vi "Filter for Classes.vi"(11 "rename data":T2) -> (1 "found classes?":bool, 3 "renamed classes":T1[](array[typedef]))   [LabVIEW 2021, in "MeasurementService Editor.lvlib"]
uses:
  MeasurementService Editor.lvlib
  Rename Refactor Data.ctl
  Rename Refactor Mapping Info.ctl
  Rename String Mapping.ctl
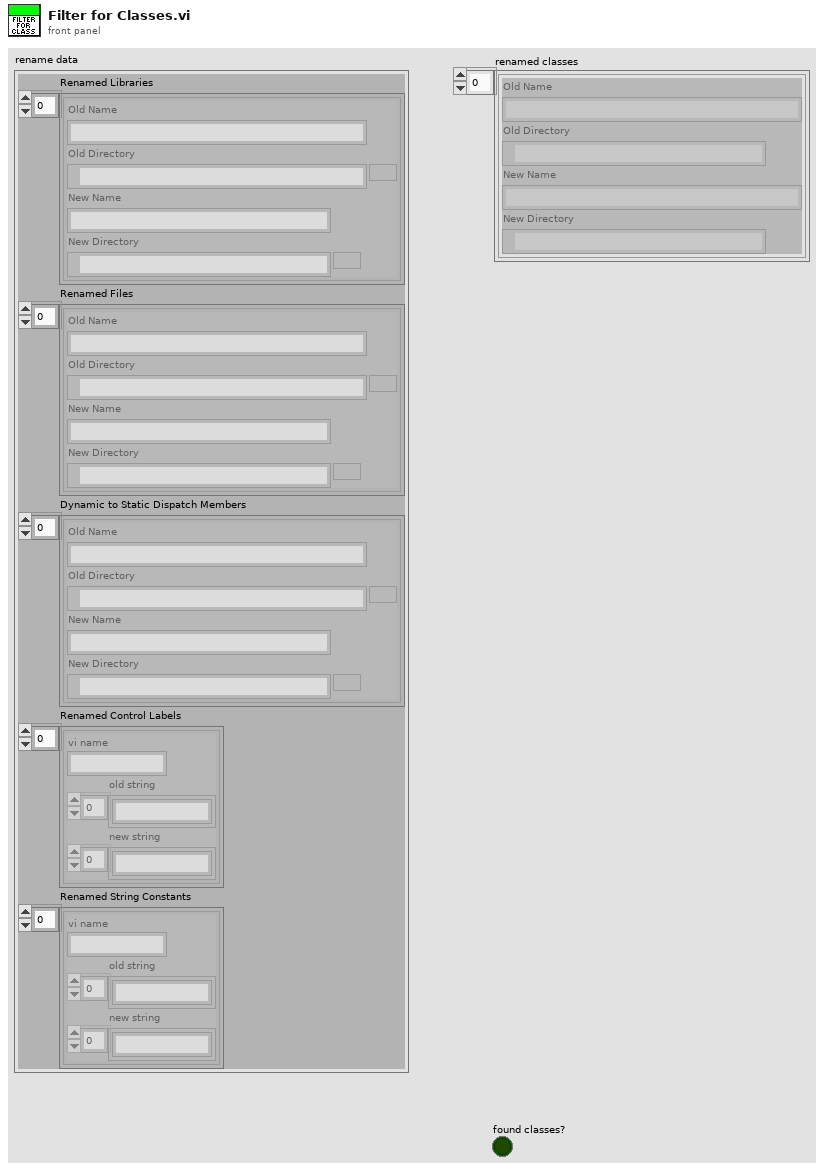
[diagram p1: front panel]
types:
  T1 = typedef "MeasurementService Editor.lvlib/Rename Refactor Mapping Info.ctl" = cluster{"Old Name":string, "Old Directory":path, "New Name":string, "New Directory":path}
  T2 = typedef "MeasurementService Editor.lvlib/Rename Refactor Data.ctl" = cluster{"Renamed Libraries":T1[], "Renamed Files":T1[], "Dynamic to Static Dispatch Members":T1[], "Renamed Control Labels":T3[], "Renamed String Constants":T3[]}
  T3 = typedef "MeasurementService Editor.lvlib/Rename String Mapping.ctl" = cluster{"vi name":string, "old string":string[], "new string":string[]}
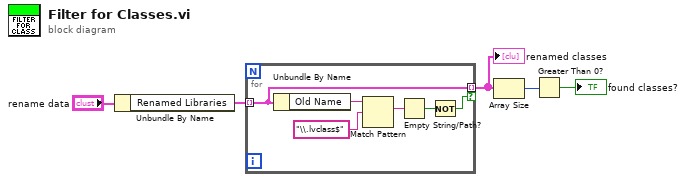
[diagram p0: block diagram]
diagram:
  n1 = Unbundle By Name("rename data") -> ("Renamed Libraries"=w4:T1[])
  n2 = for {
    tunnel: w4 -> [w7] mode=indexing
    tunnel: [w7] -> w3 mode=indexing if=w6
    n3 = Unbundle By Name(w7) -> ("Old Name"=w11:string)
    n4 = Match Pattern(string=w11, regular expression="\\.lvclass$") -> (match substring=w9:string)  [unwired: 1 in, 3 out]
    n5 = Empty String/Path?(string/path=w9) -> (empty?=w8:bool)
    n6 = Not(x=w8) -> (.not. x?=w6:bool)
  }
  "renamed classes" <- w3
  n7 = Array Size(array=w3) -> (size(s)=w2:i32)
  n8 = Greater Than 0?(x=w2) -> (x > 0?=→"found classes?":bool)
